vi "Swerve_Set.vi"(2 "Port (Port A)":i32(ring) items=["Port A", "Port B", "Port C", "Port D"], 3 "NXT/EV3":T1, 4 "Intended Angle":i32, 9 "Wait? (T)":bool=TRUE) -> (0 "NXT/EV3":T1)   [LabVIEW 2012]
uses:
  <vilib>/NXT/Subs/LVHSConnector.ctl
  <vilib>/NXT/LegoClasses/BrickReference/BrickReference.lvclass
  CLIB/CThread/Core/CThread Thread Properties.ctl
  CLIB/CRef/Core/Master Types.ctl
  CLIB/CRef/LabelCore/CRefLabel Static Reference.vi
  CLIB/CThread/Base/CThread Base - VI Reference.vi
  CLIB/CRef/Interface/CRef Numeric.llb/CRef Set I32.vi
  CLIB/CThread/Base/CThread Base - While Loop.vi
  CLIB/CThread/Base/CThread Base - Get Execution State.vi
  CLIB/CRef/XNodes/labelnode/CRef Label Node.xnode
  CLIB/CThread/XNodes/referencenode/CThread VI Reference.xnode
  CLIB/CThread/XNodes/terminalnode/CThread VI Terminal Node.xnode
  CLIB/CRef/Interface/CRef Boolean.llb/Boolean CReference.ctl
  CLIB/CRef/Interface/CRef Numeric.llb/I32 CReference.ctl
  CLIB/CRef/CRef.lvlib
  CLIB/CThread/CThread.lvlib
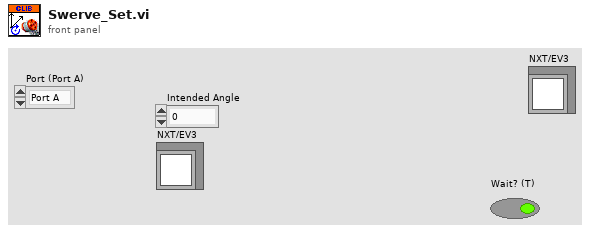
[diagram p1: front panel]
types:
  T1 = typedef "LVHSConnector.ctl" = refnum<class "BrickReference.lvclass">
  T2 = typedef "CThread.lvlib/CThread Thread Properties.ctl" = cluster{"Post-Run Delay (5ms)":u32}
  T3 = cluster{"Boolean CRef Address":u16, "Type":enum8{"Null", "Boolean", "U8", "I8", "U16", "I16", "U32", "I32", "U64", "I64", "Single", "Double", "Extended", "CSG", "CDB", "CXT", "Boolean(Def)"}}
  T4 = typedef "CRef.lvlib/Boolean CReference.ctl" = cluster{"Boolean CRef Address":u16, "Type":enum8{"Null", "Boolean", "U8", "I8", "U16", "I16", "U32", "I32", "U64", "I64", "Single", "Double", "Extended", "CSG", "CDB", "CXT", "Boolean(Def)"}}
  T5 = enum16{"Inactive", "While Loop", "For Loop", "Do When Loop", "Scheduled"}
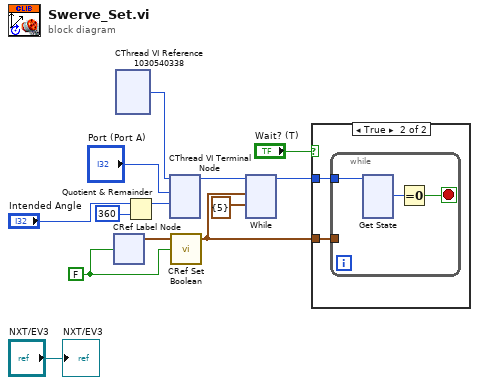
[diagram p0: block diagram]
diagram:
  w4 = FALSE ("Initial Value (if creating)")
  n1 = xnode "CRef Label Node"("Initial Value (if creating)"=w4) -> ("Boolean CReference"=w6:T3)  [unwired: 2 out]
  n2 = xnode "CThread VI Reference 1030540338"() -> ("Swerve_Slave.vi"=w2:i32)
  n3 = Quotient & Remainder(x="Intended Angle", y=360) -> (x-y*floor(x/y)=w8:i32)  [unwired: 1 out]
  n4 = xnode "CThread VI Terminal Node"("CLIB VI Reference"=w2, "PortIn"="Port (Port A)", "Intended Angle"=w8) -> ("Swerve_Slave.vi"=w12:i32)
  n5 = call "CRef Set Boolean.vi"("Value"=w4, "Boolean CReference"=w6) -> ("Boolean CReference"=w5:T4)  [unwired: 3 in]
  n6 = xnode "While"("CLIB VI Reference"=w12, "Thread Properties"=T2 {"Post-Run Delay (5ms)"=5}, "CRef: Conditional Terminal"=w5) -> ("Swerve_Slave.vi"=w3:i32)  [unwired: 1 out]
  n7 = case shown="True" "Wait? (T)" {
    tunnel: w5 -> [_ w15]
    tunnel: w3 -> [_ w14]
    frame False {
    }
    frame True {
      n8 = while {
        tunnel: w15 -> [_]
        tunnel: w14 -> [w16]
        stop <- w17 stop-if-true
        n9 = xnode "Get State"("CLIB VI Reference"=w16) -> ("Action"=w18:T5)  [unwired: 3 out]
        n10 = Equal To 0?(x=w18) -> (x = 0?=w17:bool)
      }
    }
  }
  "NXT/EV3" <- "NXT/EV3"
